vi "Extract Newest Using Moving Pointer.vi"(6 "Create if not found":bool=TRUE, 7 "Pointer Index":i32=-1, 8 "Error":errorcluster, 9 "Moving Pointer":refnum<class "_Pointer.lvclass">, 11 "WavBuf":refnum<class "WavBuf.lvclass">) -> (0 "Error Out":errorcluster, 1 "Moving Pointer Out":refnum<class "_Pointer.lvclass">, 2 "Newest Data Out":T1, 3 "WavBuf Out":refnum<class "WavBuf.lvclass">, 5 "Pointer Index Out":i32)   [LabVIEW 2020, in "WavBuf.lvclass"]
uses:
  WavBuf.lvclass
  Universal Controls/Waveform_Data.ctl
  Pointer/_Pointer.lvclass
  WavBuf.lvclass/WavBuf.ctl
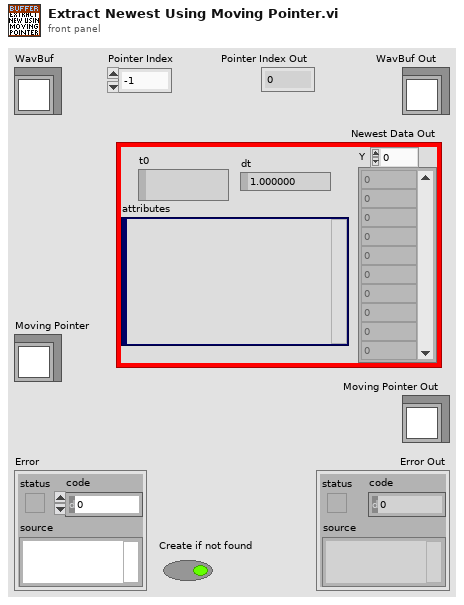
[diagram p1: front panel]
types:
  T1 = typedef "Waveform_Data.ctl" = waveform(dbl)
  T2 = typedef "Ref_DVR_Buffer.ctl" = refnum<data-value>
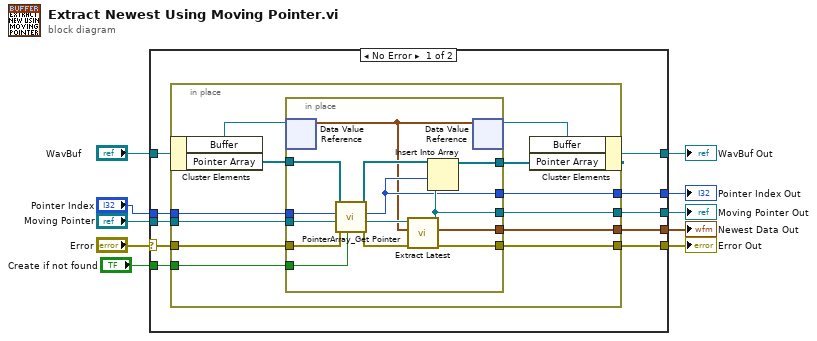
[diagram p0: block diagram]
diagram:
  n1 = case shown="No Error" "Error" {
    selector: "Error" -> [w18 w49]
    tunnel: [w17 w49] -> w9
    tunnel: [w19 w48] -> w7
    tunnel: "WavBuf" -> [w20 w48]
    tunnel: [w16 _] -> w6
    tunnel: "Moving Pointer" -> [w15 w47]
    tunnel: "Pointer Index" -> [w14 _]
    tunnel: [w13 w47] -> w3
    tunnel: [w12 _] -> w2
    tunnel: "Create if not found" -> [w11 _]
    frame No Error {
      n2 = in-place {
        in-place-border: w18 -> [w32]
        in-place-border: [w27] -> w17
        in-place-border: [w26] -> w16
        in-place-border: w15 -> [w29]
        in-place-border: w14 -> [w28]
        in-place-border: [w25] -> w13
        in-place-border: [w24] -> w12
        in-place-border: w11 -> [w23]
        n3 = in-place-cluster #1(w20) -> ("Buffer"=w22:T2, "Pointer Array"=w31:refnum<class "_Pointer.lvclass">[])
        n4 = in-place {
          in-place-border: w32 -> [w46]
          in-place-border: w31 -> [w44]
          in-place-border: [w43] -> w30
          in-place-border: w29 -> [w42]
          in-place-border: w28 -> [w41]
          in-place-border: [w39] -> w27
          in-place-border: [w37] -> w26
          in-place-border: [w36] -> w25
          in-place-border: [w35] -> w24
          in-place-border: w23 -> [w34]
          n5 = in-place-dvr #2(w22) -> (w33:T1)  [unwired: 1 out]
          n6 = call "PointerArray_Get Pointer.vi"("Create If Not Found"=w34, "Error"=w46, "Pointer"=w42, "Index"=w41, "Pointer Array"=w44) -> ("Error Out"=w40:errorcluster, "Pointer Out"=w38:refnum<class "_Pointer.lvclass">, "Index Out"=w35:i32, "Pointer Array Out"=w45:refnum<class "_Pointer.lvclass">[])  [unwired: 2 in, 1 out]
          n7 = call-dynamic "Extract Latest.vi"("Error"=w40, "Raw Data Waveform"=w33, "((Pointer))"=w38) -> ("Error Out"=w39:errorcluster, "Waveform Out"=w37:T1, "((Pointer)) Out"=w36:refnum<class "_Pointer.lvclass">)  [unwired: 6 in]
          n8 = Insert Into Array(array=w45, index=w35, new element=w36) -> (w43:refnum<class "_Pointer.lvclass">[])
          n9 = in-place-dvr #2(w33) -> (w21:T2)  [unwired: 1 out]
        }
        n10 = in-place-cluster #1("Buffer"=w21, "Pointer Array"=w30) -> (w19:refnum<class "WavBuf.lvclass">)
      }
    }
    frame Error {
    }
  }
  "Error Out" <- w9
  "WavBuf Out" <- w7
  "Newest Data Out" <- w6
  "Moving Pointer Out" <- w3
  "Pointer Index Out" <- w2
